vi "AD2_DO_SDK_Init.vi"(0 "object in":refnum<class "AD2_DO_SDK.lvclass">, 2 "phdwf":i32, 5 "error in (no error)":errorcluster) -> (14 "object out":refnum<class "AD2_DO_SDK.lvclass">, 19 "error out":errorcluster)   [LabVIEW 2023, in "AD2_DO_SDK.lvclass"]
uses:
  AD2_DO_SDK.lvclass
  AD2_DO_SDK.lvclass/AD2_DO_SDK.ctl
  DOSingleCh.ctl
  Olasdwf/Olasdwf.lvlib
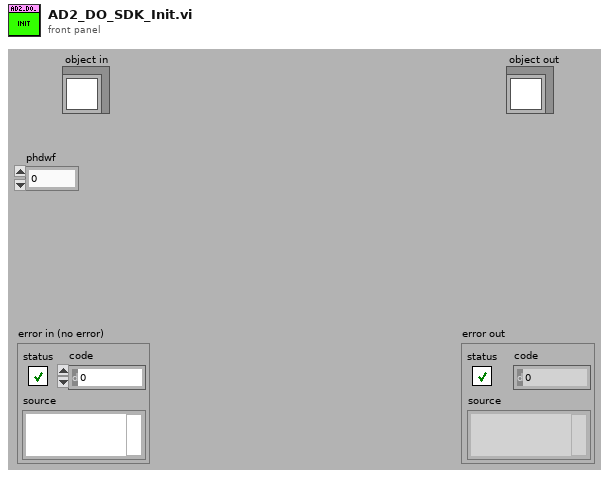
[diagram p1: front panel]
types:
  T1 = typedef "AD2_DO_SDK.lvclass/DOSingleCh.ctl" = cluster{"Ch Index":i32, "Enable":bool, "Clock DIvider":u32, "Type":i32, "DigitalOutOutput":u16, "IdleState":u16, "CounterData":cluster{"NoHighBits":u32, "NoLowBits":u32, "NoInitialBits":u32, "Start High":bool}, "Custom Data":cluster{"countOfBits":u32, "rgBits":u8[]}}
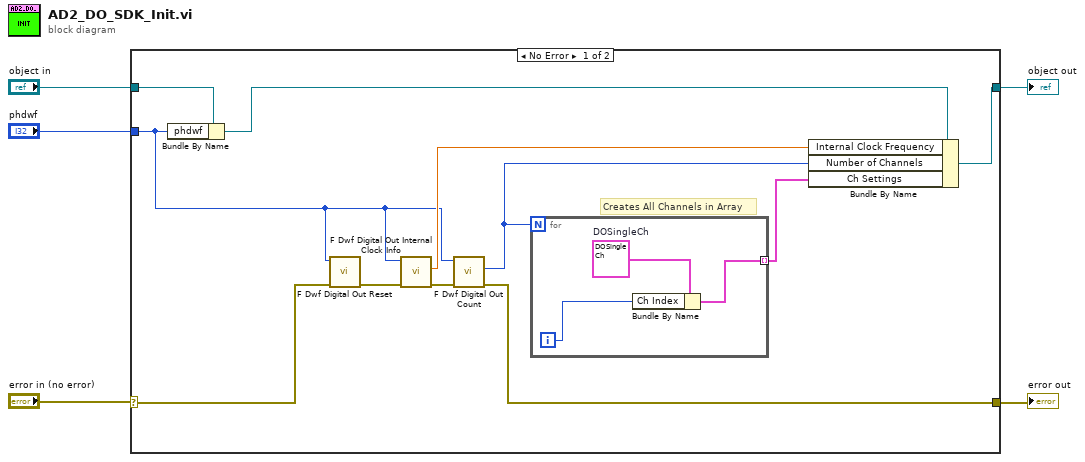
[diagram p0: block diagram]
diagram:
  n1 = case shown="No Error" "error in (no error)" {
    selector: "error in (no error)" -> [w7 w20]
    tunnel: "object in" -> [w13 w21]
    tunnel: [w16 w21] -> w4
    tunnel: [w11 w20] -> w2
    tunnel: "phdwf" -> [w8 _]
    frame No Error {
      # "Creates All Channels in Array"
      n2 = Bundle By Name(cluster=w13, "phdwf"=w8) -> (w14:refnum<class "AD2_DO_SDK.lvclass">)
      n3 = call "F Dwf Digital Out Reset.vi"("error in (no error)"=w7, "hdwf"=w8) -> ("error out"=w6:errorcluster)  [unwired: 8 in, 1 out]
      n4 = call "F Dwf Digital Out Internal Clock Info.vi"("error in (no error)"=w6, "hdwf"=w8) -> ("error out"=w12:errorcluster, "phzFreq out"=w15:dbl)  [unwired: 7 in, 1 out]
      n5 = call "F Dwf Digital Out Count.vi"("error in (no error)"=w12, "hdwf"=w8) -> ("error out"=w11:errorcluster, "pcChannel out"=w10:i32)  [unwired: 7 in, 1 out]
      n6 = for {
        N: w10 -> [_]
        tunnel: [w17] -> w9 mode=indexing
        i -> [w18]
        w19 = T1 {"Ch Index"=0, "Enable"=FALSE, "Clock DIvider"=0, "Type"=0, "DigitalOutOutput"=0, "IdleState"=0, "CounterData"={"NoHighBits"=0, "NoLowBits"=0, "NoInitialBits"=0, "Start High"=FALSE}, "Custom Data"={"countOfBits"=0, "rgBits"=[]}}  # DOSingleCh
        n7 = Bundle By Name(cluster=w19, "Ch Index"=w18) -> (w17:T1)
      }
      n8 = Bundle By Name(cluster=w14, "Internal Clock Frequency"=w15, "Number of Channels"=w10, "Ch Settings"=w9) -> (w16:refnum<class "AD2_DO_SDK.lvclass">)
    }
    frame Error {
    }
  }
  "object out" <- w4
  "error out" <- w2
